vi "create_l3_batch.vi"   [LabVIEW 2015, in "lv-builder-l3.lvlib"]
uses:
  lv-builder-l3.lvlib
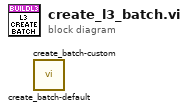
[diagram p0: block diagram]
diagram:
  n1 = call "create_batch-default.vi"() -> ()  [unwired: 10 in, 2 out]
  n2 = call "create_batch-custom.vi"() -> ()  [unwired: 10 in, 2 out]
